vi "Write Slot Length (s).vi"(8 "error in (no error)":errorcluster, 10 "Slot Length (s)":dbl=0.0001 format="%.3p", 11 "SPECAN_IQSLOT in":refnum<class "SPECAN_IQSLOT.lvclass">) -> (0 "error out":errorcluster, 3 "SPECAN_IQSLOT out":refnum<class "SPECAN_IQSLOT.lvclass">)   [LabVIEW 2018, in "SPECAN_IQSLOT.lvlib" / "SPECAN_IQSLOT.lvclass"]
uses:
  SPECAN_IQSLOT.lvclass
  SPECAN_IQSLOT.lvclass/SPECAN_IQSLOT.ctl
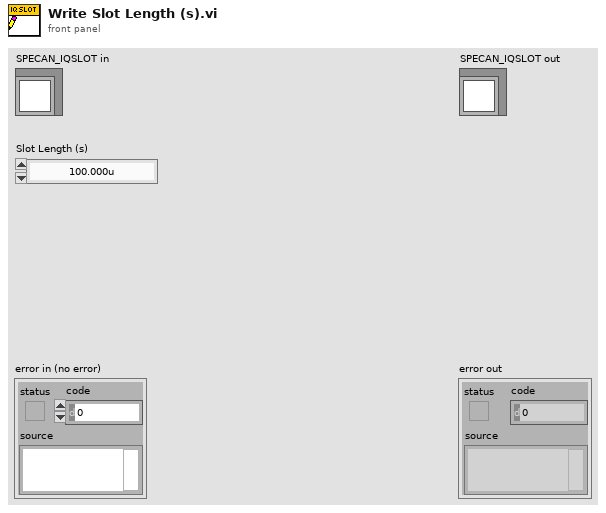
[diagram p1: front panel]
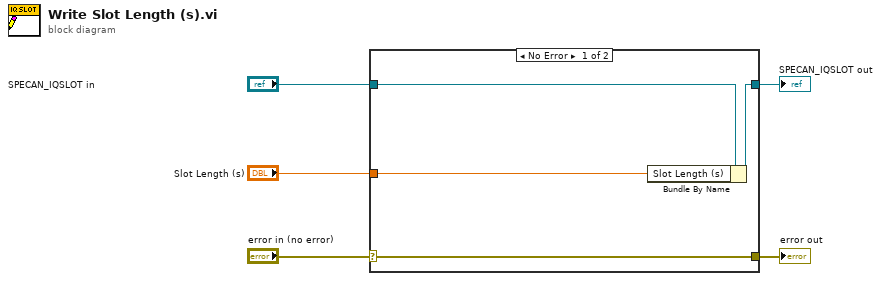
[diagram p0: block diagram]
diagram:
  n1 = case shown="No Error" "error in (no error)" {
    selector: "error in (no error)" -> [w9 w10]
    tunnel: [w9 w10] -> w4
    tunnel: [w7 w11] -> w2
    tunnel: "SPECAN_IQSLOT in" -> [w8 w11]
    tunnel: "Slot Length (s)" -> [w6 _]
    frame No Error {
      n2 = Bundle By Name(cluster=w8, "Slot Length (s)"=w6) -> (w7:refnum<class "SPECAN_IQSLOT.lvclass">)
    }
    frame Error {
    }
  }
  "error out" <- w4
  "SPECAN_IQSLOT out" <- w2
